vi "Read Analog Input.vi"(0 "VISA Refnum in":refnum<visa-resource-name>, 5 "#Pin analogico":enum16{"AI-0", "AI-1", "AI-2", "AI-3"}(ring), 7 "Vref Máx":i32, 9 "Resolucion ADC Bits":i32, 11 "error in (no error)":errorcluster) -> (4 "VISA Refnum out":refnum<visa-resource-name>, 8 "Volt":dbl, 15 "error out":errorcluster)   [LabVIEW 2020, in "Hardware DAQ.lvlib"]
uses:
  Hardware DAQ.lvlib
panel:
  out "resulting string":string
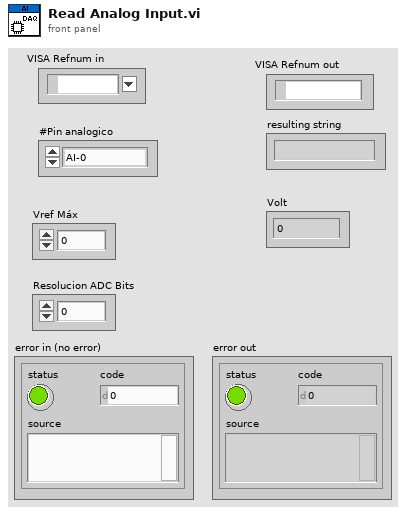
[diagram p1: front panel]
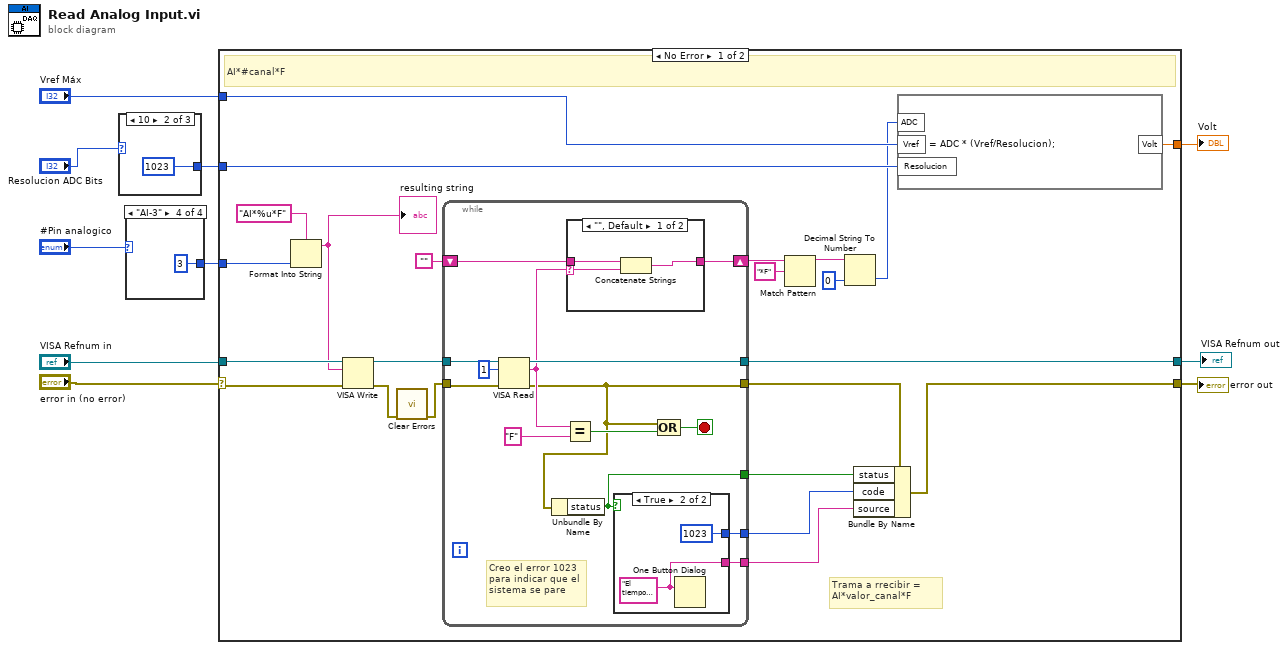
[diagram p0: block diagram]
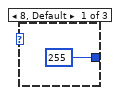
[diagram p2: hidden frame]
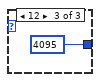
[diagram p3: hidden frame]
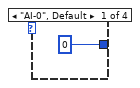
[diagram p4: hidden frame]
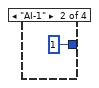
[diagram p5: hidden frame]
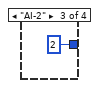
[diagram p6: hidden frame]
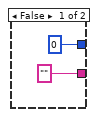
[diagram p7: hidden frame]
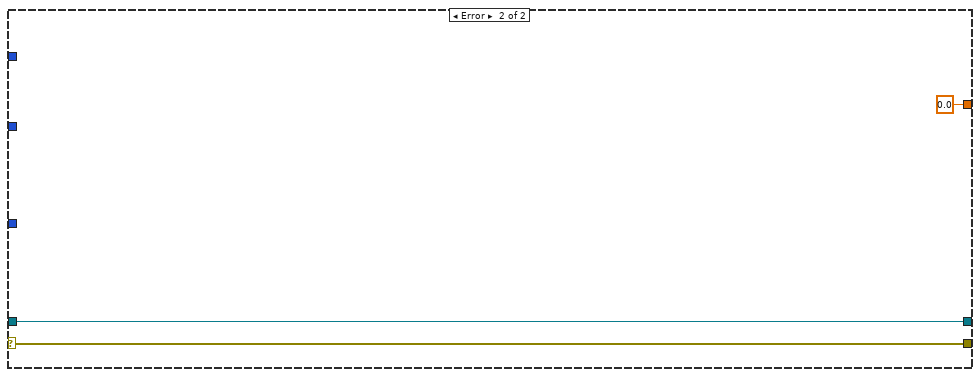
[diagram p9: hidden frame]
diagram:
  n1 = case shown="10" "Resolucion ADC Bits" {
    tunnel: [255 ("Resolucion ADC Bits") 1023 ("Resolucion ADC Bits") 4095 ("Resolucion ADC Bits")] -> w1
    frame 8, Default {
    }
    frame 10 {
    }
    frame 12 {
    }
  }
  n2 = case shown="\"AI-3\"" "#Pin analogico" {
    tunnel: [u32 0 ("input 1") u32 1 ("input 1") u32 2 ("input 1") u32 3 ("input 1")] -> w3
    frame "AI-0", Default {
    }
    frame "AI-1" {
    }
    frame "AI-2" {
    }
    frame "AI-3" {
    }
  }
  n3 = case shown="No Error" "error in (no error)" {
    selector: "error in (no error)" -> [w40 w65]
    tunnel: [w20 w65] -> w9
    tunnel: "VISA Refnum in" -> [w39 w63]
    tunnel: [w36 w63] -> w7
    tunnel: "Vref Máx" -> [w34 _]
    tunnel: w1 -> [w33 _]
    tunnel: [w27 0.0 ("Volt")] -> w5
    tunnel: w3 -> [w25 _]
    frame No Error {
      # "Trama a rrecibir =     \nAI*valor_canal*F"
      # "AI*#canal*F"
      n4 = Format Into String(format string="AI*%u*F", w25) -> (resulting string=w24:string)  [unwired: 2 in, 1 out]
      "resulting string" <- w24
      n5 = VISA Write(VISA resource name=w39, write buffer=w24, error in (no error)=w40) -> (VISA resource name out=w37:refnum<visa-resource-name>, error out=w38:errorcluster)  [unwired: 1 out]
      n6 = call <vilib>:"Clear Errors.vi"("error in (no error)"=w38) -> ("error out"=w23:errorcluster)  [unwired: 5 in, 1 out]
      n7 = while {
        tunnel: [w42] -> w22
        tunnel: w23 -> [w53]
        tunnel: w37 -> [w54]
        tunnel: [w51] -> w36
        shift-right: [w49] -> w32
        shift-left: "" -> [w50]
        tunnel: [w44] -> w21
        tunnel: [w43] -> w19
        tunnel: [w41] -> w18
        stop <- w45 stop-if-true
        # "Creo el error 1023\npara indicar que el\nsistema se pare"
        n8 = VISA Read(VISA resource name=w54, byte count=u32 1, error in (no error)=w53) -> (VISA resource name out=w51:refnum<visa-resource-name>, read buffer=w48:string, error out=w42:errorcluster)  [unwired: 1 out]
        n9 = Unbundle By Name(w42) -> ("status"=w41:bool)
        n10 = Equal?(x=w48, y="F") -> (x = y?=w46:bool)
        n11 = case shown="\"\", Default" w48 {
          selector: w48 -> [w59 _]
          tunnel: w50 -> [w61 w62]
          tunnel: [w60 w62] -> w49
          frame "", Default {
            n12 = Concatenate Strings(w61, w59) -> (w60:string)
          }
          frame "*", "A", "F", "I" {
          }
        }
        n13 = case shown="True" w41 {
          tunnel: ["" ("message") w57] -> w44
          tunnel: [0 ("code") 1023 ("code")] -> w43
          frame False {
          }
          frame True {
            w57 = "El tiempo de espera ha excedido\nal momento de leer datos del hardware" ("message")
            n14 = One Button Dialog(message=w57) -> ()  [unwired: 1 in, 1 out]
          }
        }
        n15 = Compound Arithmetic op=OR(w42, w46) -> (w45:bool)
      }
      n16 = Match Pattern(string=w32, regular expression="*F") -> (before substring=w30:string)  [unwired: 1 in, 3 out]
      n17 = Decimal String To Number(string=w30, default (0L)=u16 0 ("default (0 I32)")) -> (number=w28:u16)  [unwired: 1 in, 1 out]
      n18 = Bundle By Name(cluster=w22, "status"=w18, "code"=w19, "source"=w21) -> (w20:errorcluster)
      n19 = formula code="Volt = ADC * (Vref/Resolucion);"("Vref"=w34, "Resolucion"=w33, "ADC"=w28) -> ("Volt"=w27:dbl)
    }
    frame Error {
    }
  }
  "error out" <- w9
  "VISA Refnum out" <- w7
  "Volt" <- w5
